vi "RT Error Handler - RSI Low Speed.vi"(8 "error in (no error)":errorcluster, 11 "Message Queue":refnum<queue>) -> (2 "Enqueued Error?":bool, 3 "dup Message Queue":refnum<queue>)   [LabVIEW 2018]
uses:
  support/Message Queue/Message Cluster.ctl
  support/Message Queue/Message Queue.lvlib
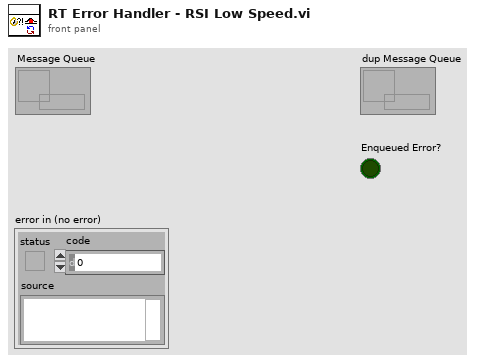
[diagram p1: front panel]
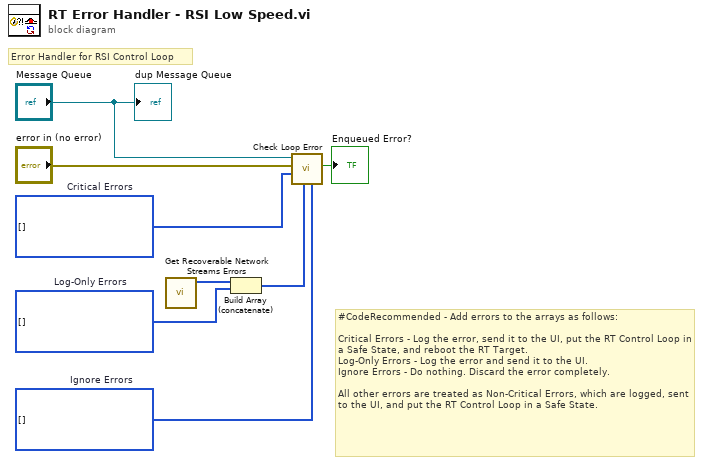
[diagram p0: block diagram]
diagram:
  w7 = i32[] []  # Ignore Errors
  w3 = i32[] []  # Log-Only Errors
  w8 = i32[] []  # Critical Errors
  # "#CodeRecommended - Add errors to the arrays as follows:\n\nCritical Errors - Log the error, send it to the UI, put the RT Control Loop in a Safe State, and reboot the RT Target.\nLog-Only Errors - Log the error and send it to the UI.\nIgnore Errors - Do nothing. Discard the error completely.\n\nAll other errors are treated as Non-Critical Errors, which are logged, sent to the UI, and put the RT Control Loop in a Safe State."
  # "Error Handler for RSI Control Loop"
  n1 = call "Get Recoverable Network Streams Errors.vi"() -> ("recoverable network streams errors"=w4:i32[])  [unwired: 11 in]
  n2 = Build Array (concatenate)(w4, w3) -> (w2:i32[])
  n3 = call "Check Loop Error.vi"("Ignore Errors"=w7, "Log-Only Errors"=w2, "Critical Errors"=w8, "error to process"="error in (no error)", "Message Queue"="Message Queue") -> ("Enqueued Error?"=→"Enqueued Error?":bool)  [unwired: 5 in, 1 out]
  "dup Message Queue" <- "Message Queue"
